vi "Fetch Multiple Record Multiple Channel (I16).vi"(5 "FIFO Type":T1=enum."Fast FIFO", 7 "Timeout (s)":i32=5, 8 "error in":errorcluster, 10 "Records to Fetch":i32, 11 "FPGA VI Reference In":refnum<k20>) -> (0 "error out":errorcluster, 2 "Acquired Data":i16[][](array[numeric]), 3 "FPGA VI Reference Out":refnum<k20>, 4 "Elements Remaining":u32)   [LabVIEW 2012]
uses:
  <userlib>/FlexRIO Host Library/FlexRIO Host API/Acquire/FIFO Type.ctl
  <userlib>/FlexRIO Host Library/FlexRIO Host API/Acquire/Fetch/Fetch Acquired Data (I16).vi
  <vilib>/Utility/error.llb/Error Cluster From Error Code.vi
  <vilib>/rvi/errors/niLvFpgaAdjustHostInterfaceError.vi
  <vilib>/rvi/interface/nirviReadWriteControl/nirviReadWriteControl.xnode
  NiFpgaLv.dll
  <vilib>/rvi/interface/Simulation/niFpgaSimulationCallBeginRW.vi
  <userlib>/FlexRIO Host Library/FlexRIO Host Library (User).lvlib
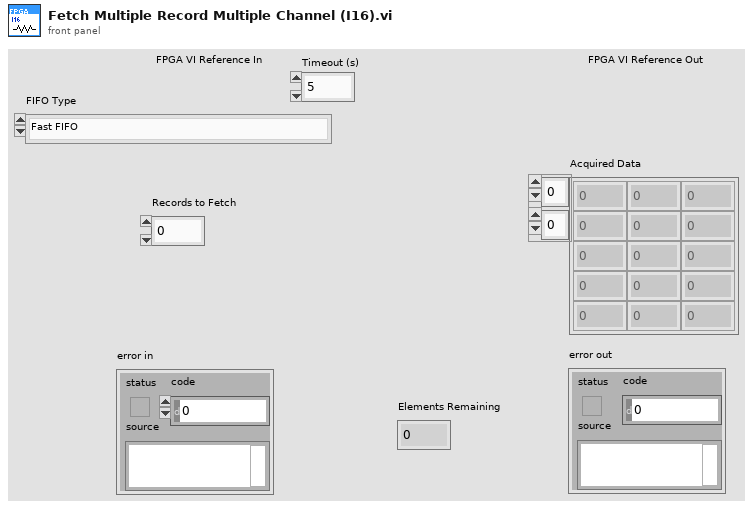
[diagram p1: front panel]
types:
  T1 = typedef "FIFO Type.ctl" = enum16{"FPGA to Host FIFO (U64)", "Generic", "FPGA to Host FIFO (U32)", "Fast FIFO"}
  T2 = cluster{"Load Record Parameters?":bool, "Pre Trigger Samples":u16, "Samples per Record":u16, "Trigger Hold Off":u16, "Record Count":u16}
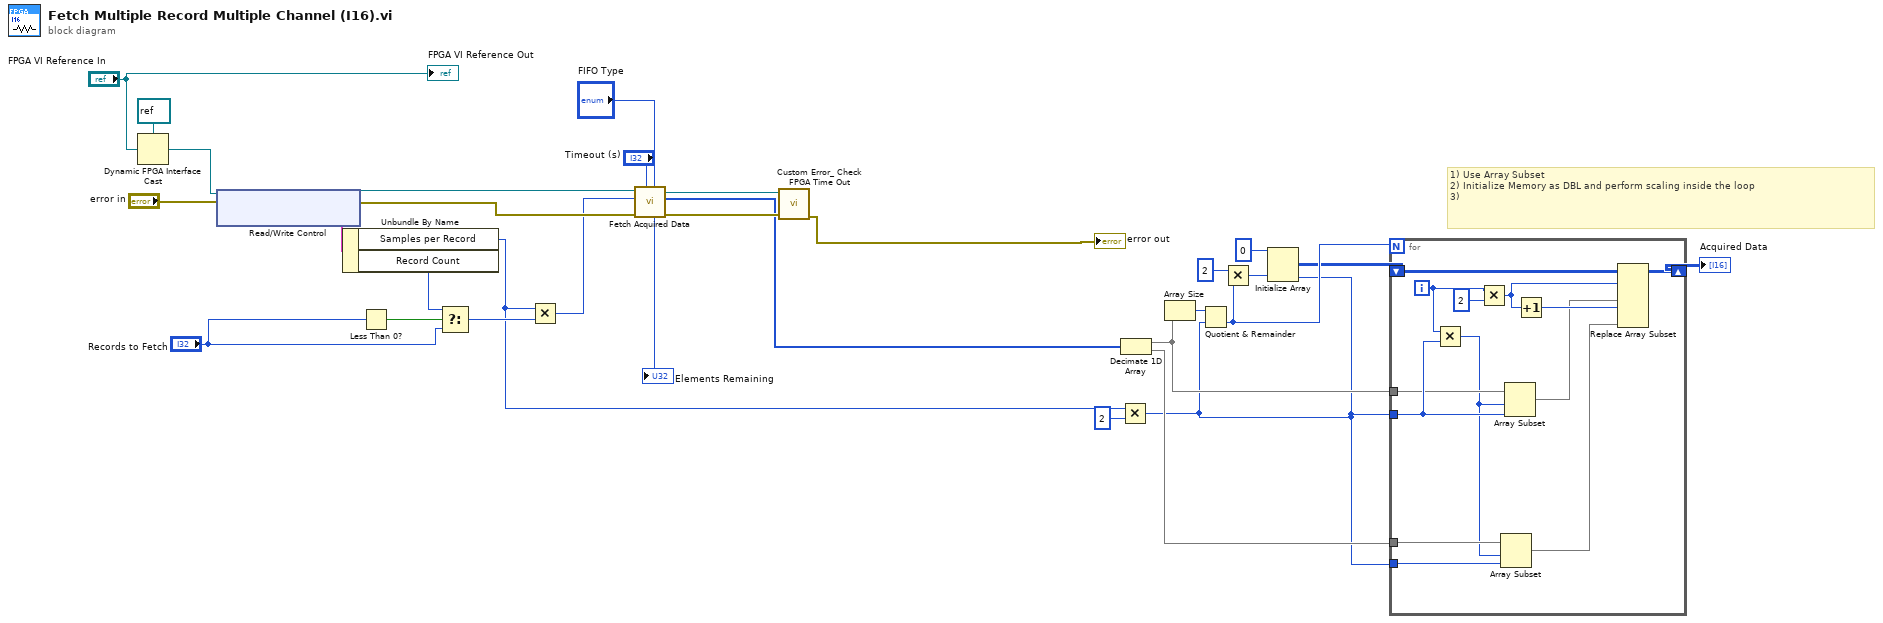
[diagram p0: block diagram]
diagram:
  # "1) Use Array Subset\n2) Initialize Memory as DBL and perform scaling inside the loop\n3)"
  n1 = Dynamic FPGA Interface Cast(Session In=refnum<k20> refnum ("Type"), Type="FPGA VI Reference In") -> (Session Out=w28:refnum<k20>)
  n2 = xnode "Read/Write Control"("FPGA VI Reference In"=w28, "error in"="error in") -> ("FPGA VI Reference Out"=w23:refnum<k20>, "error out"=w22:errorcluster, "Record Parameters"=w27:T2)
  n3 = Unbundle By Name(w27) -> ("Samples per Record"=w17:u16, "Record Count"=w25:u16)
  n4 = Less Than 0?(x="Records to Fetch") -> (x < 0?=w26:bool)
  n5 = Select(t=w25, s=w26, f="Records to Fetch") -> (s? t:f=w18:i32)
  n6 = Multiply(x=w17, y=w18) -> (x*y=w21:i32)
  n7 = call-poly <userlib>:"Fetch Acquired Data.vi"("FIFO Type"="FIFO Type", "Timeout (s)"="Timeout (s)", "error out"=w22, "Samples"=w21, "FPGA Reference In"=w23) -> ("error out"=w12:errorcluster, "Data"=w1:i16[], "FPGA Reference Out"=w13:refnum<k20>, "Elements Remaining"=→"Elements Remaining":u32)  [unwired: 3 in]
  n8 = call <userlib>:"Custom Error_ Check FPGA Time Out.vi"("error in"=w12, "FPGA VI Reference In"=w13) -> ("error out"=→"error out":errorcluster)  [unwired: 8 in, 1 out]
  n9 = Multiply(x=w17, y=u16 2) -> (x*y=w5:u16)
  n10 = Decimate 1D Array(w1) -> (w15:i16[], w6:i16[])
  n11 = Array Size(array=w15) -> (size(s)=w14:i32)
  n12 = Quotient & Remainder(x=w14, y=w5) -> (floor(x/y)=w9:i32)  [unwired: 1 out]
  n13 = Multiply(x=2, y=w9) -> (x*y=w10:i32)
  n14 = Initialize Array(i16 0 ("element"), w10, w5) -> (w7:i16[][])
  n15 = for {
    N: w9 -> [_]
    tunnel: w15 -> [w43]
    tunnel: w5 -> [w44]
    tunnel: w6 -> [w42]
    tunnel: w5 -> [w40]
    shift-right: [w38] -> w4
    shift-left: w7 -> [w39]
    i -> [w37]
    n16 = Multiply(x=w37, y=w44) -> (x*y=w41:i32)
    n17 = Multiply(x=w37, y=2) -> (x*y=w35:i32)
    n18 = Array Subset(array=w42, index=w41, length=w40) -> (w32:i16[])
    n19 = Array Subset(array=w43, index=w41, length=w44) -> (w33:i16[])
    n20 = Increment(x=w35) -> (x+1=w34:i32)
    n21 = Replace Array Subset(array=w39, new element #1=w33, index (row) #1=w35, new element #2=w32, index (row) #2=w34) -> (w38:i16[][])  [unwired: 2 in]
  }
  "Acquired Data" <- w4
  "FPGA VI Reference Out" <- "FPGA VI Reference In"
